vi "UT--Parse URIs.vi"() -> (3 "Test Passed?":bool)   [LabVIEW 2017]
doc: "Self-checking test VI in the URI palette. It round-trips a set of URIs through Parse URI and reports Test Passed?."
uses:
  URI.lvlib
panel:
  out "Test Results":T1
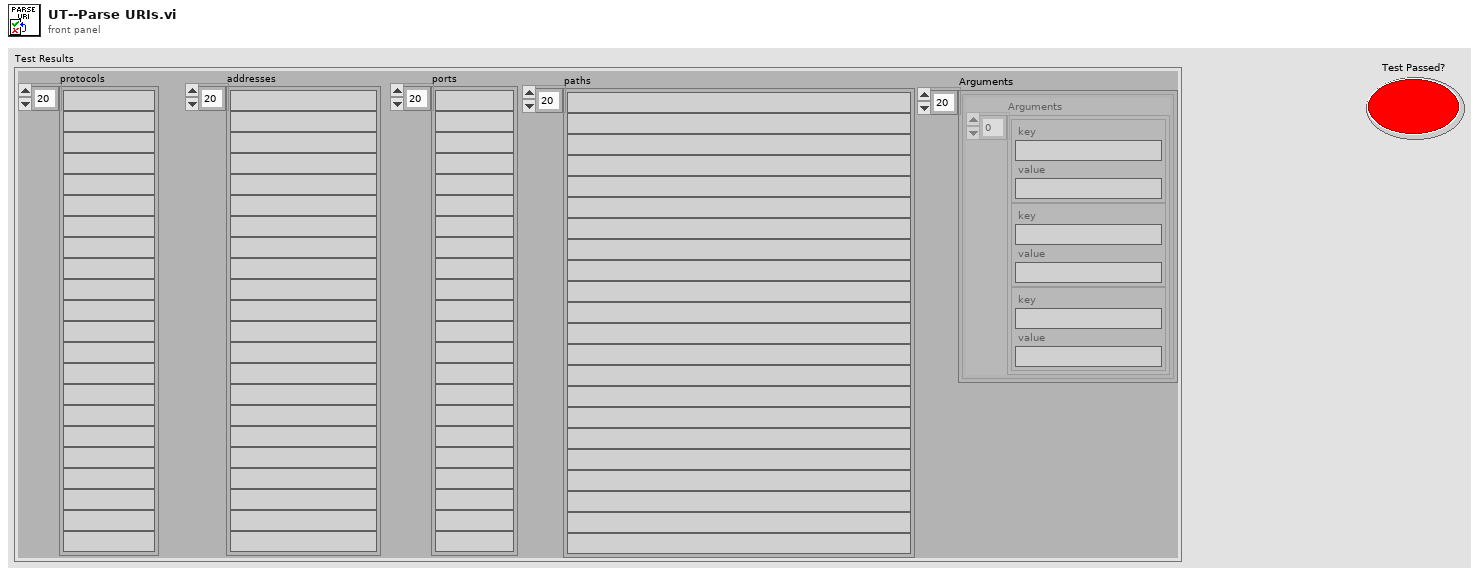
[diagram p1: front panel]
types:
  T1 = cluster{"protocols":string[], "addresses":string[], "ports":string[], "paths":string[], "Arguments":cluster{"Arguments":cluster{"key":string, "value":string}[]}[]}
  T2 = cluster{"Arguments":cluster{"key":string, "value":string}[]}
  T3 = cluster{"protocols":bool[], "addresses":bool[], "ports":bool[], "paths":bool[], "Arguments":cluster{"Arguments":cluster{"key":bool, "value":bool}[]}[]}
  T4 = cluster{"Arguments":cluster{"key":bool, "value":bool}[]}[]
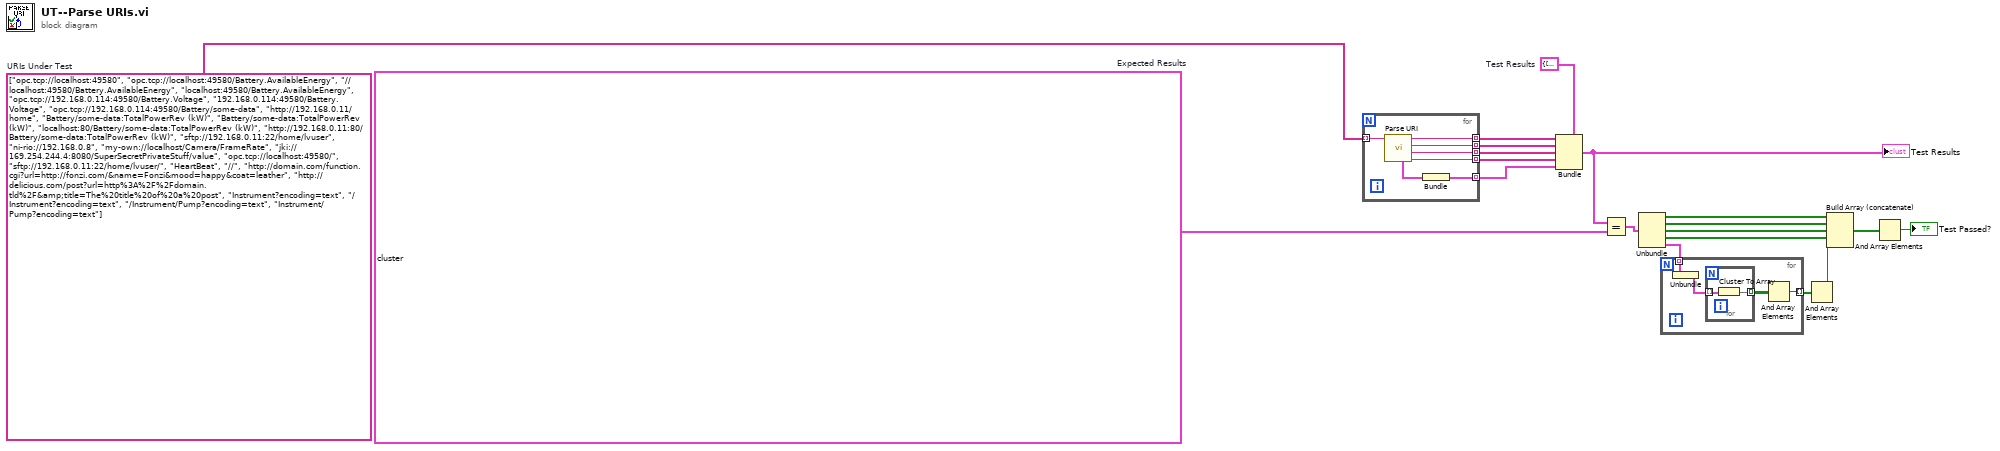
[diagram p0: block diagram]
diagram:
  w13 = T1 {"protocols"=["opc.tcp", "opc.tcp", "", "", "opc.tcp", "", "opc.tcp", "http", "", "", "", "http", "sftp", "ni-rio", "my-own", "jki", "opc.tcp", "sftp", "", "", "http", "http", "", "", "", ""], "addresses"=["localhost", "localhost", "localhost", "localhost", "192.168.0.114", "192.168.0.114", "192.168.0.114", "192.168.0.11", "", "", "localhost", "192.168.0.11", "192.168.0.11", "192.168.0.8", "localhost", "169.254.244.4", "localhost", "192.168.0.11", "", "", "domain.com", "delicious.com", "", "", "", ""], "ports"=["49580", "49580", "49580", "49580", "49580", "49580", "49580", "", "", "", "80", "80", "22", "", "", "8080", "49580", "22", "", "", "", "", "", "", "", ""], "paths"=["", "Battery.AvailableEnergy", "Battery.AvailableEnergy", "Battery.AvailableEnergy", "Battery.Voltage", "Battery.Voltage", "Battery/some-data", "home", "Battery/some-data:TotalPowerRev (kW)", "Battery/some-data:TotalPowerRev (kW)", "Battery/some-data:TotalPowerRev (kW)", "Battery/some-data:TotalPowerRev (kW)", "home/lvuser", "", "Camera/FrameRate", "SuperSecretPrivateStuff/value", "", "home/lvuser/", "HeartBeat", "", "function.cgi", "post", "Instrument", "Instrument", "Instrument/Pump", "Instrument/Pump"], "Arguments"=[{"Arguments"=[]}, {"Arguments"=[]}, {"Arguments"=[]}, {"Arguments"=[]}, {"Arguments"=[]}, {"Arguments"=[]}, {"Arguments"=[]}, {"Arguments"=[]}, {"Arguments"=[]}, {"Arguments"=[]}, {"Arguments"=[]}, {"Arguments"=[]}, {"Arguments"=[]}, {"Arguments"=[]}, {"Arguments"=[]}, {"Arguments"=[]}, {"Arguments"=[]}, {"Arguments"=[]}, {"Arguments"=[]}, {"Arguments"=[]}, {"Arguments"=[{"key"="url", "value"="http://fonzi.com/"}, {"key"="name", "value"="Fonzi"}, {"key"="mood", "value"="happy"}, {"key"="coat", "value"="leather"}]}, {"Arguments"=[{"key"="url", "value"="http://domain.tld/"}, {"key"="title", "value"="The title of a post"}]}, {"Arguments"=[{"key"="encoding", "value"="text"}]}, {"Arguments"=[{"key"="encoding", "value"="text"}]}, {"Arguments"=[{"key"="encoding", "value"="text"}]}, {"Arguments"=[{"key"="encoding", "value"="text"}]}]}  # Expected Results
  w14 = T1 {"protocols"=[], "addresses"=[], "ports"=[], "paths"=[], "Arguments"=[]}  # Test Results
  w19 = string[] ["opc.tcp://localhost:49580", "opc.tcp://localhost:49580/Battery.AvailableEnergy", "//localhost:49580/Battery.AvailableEnergy", "localhost:49580/Battery.AvailableEnergy", "opc.tcp://192.168.0.114:49580/Battery.Voltage", "192.168.0.114:49580/Battery.Voltage", "opc.tcp://192.168.0.114:49580/Battery/some-data", "http://192.168.0.11/home", "Battery/some-data:TotalPowerRev (kW)", "Battery/some-data:TotalPowerRev (kW)", "localhost:80/Battery/some-data:TotalPowerRev (kW)", "http://192.168.0.11:80/Battery/some-data:TotalPowerRev (kW)", "sftp://192.168.0.11:22/home/lvuser", "ni-rio://192.168.0.8", "my-own://localhost/Camera/FrameRate", "jki://169.254.244.4:8080/SuperSecretPrivateStuff/value", "opc.tcp://localhost:49580/", "sftp://192.168.0.11:22/home/lvuser/", "HeartBeat", "//", "http://domain.com/function.cgi?url=http://fonzi.com/&name=Fonzi&mood=happy&coat=leather", "http://delicious.com/post?url=http%3A%2F%2Fdomain.tld%2F&amp;title=The%20title%20of%20a%20post", "Instrument?encoding=text", "/Instrument?encoding=text", "/Instrument/Pump?encoding=text", "Instrument/Pump?encoding=text"]  # URIs Under Test
  n1 = for {
    tunnel: [w26] -> w18 mode=indexing
    tunnel: [w25] -> w17 mode=indexing
    tunnel: [w24] -> w16 mode=indexing
    tunnel: [w23] -> w15 mode=indexing
    tunnel: w19 -> [w22] mode=indexing
    tunnel: [w20] -> w5 mode=indexing
    n2 = call "Parse URI.vi"("URI"=w22) -> ("path"=w23:string, "port"=w24:string, "address"=w25:string, "protocol"=w26:string, "Arguments"=w21:cluster{"key":string, "value":string}[])  [unwired: 6 in]
    n3 = Bundle("Arguments"=w21) -> (w20:T2)  [unwired: 1 in]
  }
  n4 = Bundle(cluster=w14, "protocols"=w18, "addresses"=w17, "ports"=w16, "paths"=w15, "Arguments"=w5) -> (w4:T1)
  "Test Results" <- w4
  n5 = Equal?(x=w4, y=w13) -> (x = y?=w11:T3)
  n6 = Unbundle(w11) -> ("protocols"=w10:bool[], "addresses"=w7:bool[], "ports"=w8:bool[], "paths"=w9:bool[], "Arguments"=w3:T4)
  n7 = for {
    tunnel: w3 -> [w30] mode=indexing
    tunnel: [w27] -> w2 mode=indexing
    n8 = Unbundle(w30) -> ("Arguments"=w29:cluster{"key":bool, "value":bool}[])
    n9 = for {
      tunnel: w29 -> [w32] mode=indexing
      tunnel: [w31] -> w28 mode=indexing
      n10 = Cluster To Array(cluster=w32) -> (array=w31:bool[])
    }
    n11 = And Array Elements(Boolean array=w28) -> (logical AND=w27:bool)
  }
  n12 = And Array Elements(Boolean array=w2) -> (logical AND=w1:bool)
  n13 = Build Array (concatenate)(w10, w7, w8, w9, w1) -> (w6:bool[])
  n14 = And Array Elements(Boolean array=w6) -> (logical AND=→"Test Passed?":bool)
